vi "Inverse Complex FFT.vi"(10 "shift?":bool, 11 "FFT {X}":cdb[](array[numeric])) -> (0 "error":i32, 3 "X":cdb[](array[numeric]))   [LabVIEW 2020, in "NI_AALPro.lvlib"]
doc: "Computes the inverse discrete Fourier transform (IDFT) of the input sequence <B>FFT {X}</B>. You must manually select the polymorphic instance you want to use."
uses:
  NI_AALPro.lvlib
  <resource>/lvanlys.dll
panel:
  # "Inverse Complex FFT"
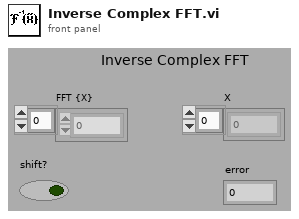
[diagram p1: front panel]
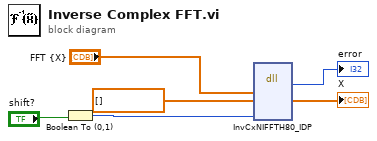
[diagram p0: block diagram]
diagram:
  n1 = Boolean To (0,1)(Boolean="shift?") -> (0, 1=w4:i16)
  n2 = dll-call lib="C:/Program Files (x86)/National Instruments/LabVIEW 2020/resource/lvanlys.*" fn="InvCxNIFFTH80_IDP"("xH"="FFT {X}", "yH"=cdb[] [] ("X"), "shift"=w4) -> ("return type"=→"error":i32, "yH"=→"X":cdb[])  [unwired: 7 in, 2 out]
